vi "Delete Cache.vi"(8 "error in (no error)":errorcluster, 11 "navX Registry Cache in":refnum<class "navX Registry Cache.lvclass">) -> (0 "error out":errorcluster, 2 "Registry Cache":u8[](array[numeric]), 3 "navX Registry Cache out":refnum<class "navX Registry Cache.lvclass">)   [LabVIEW 2015, in "navX Library v3.lvlib" / "navX Registry Cache.lvclass"]
uses:
  navX Registry Cache.lvclass
  navX Registry Cache.lvclass/navX Registry Cache.ctl
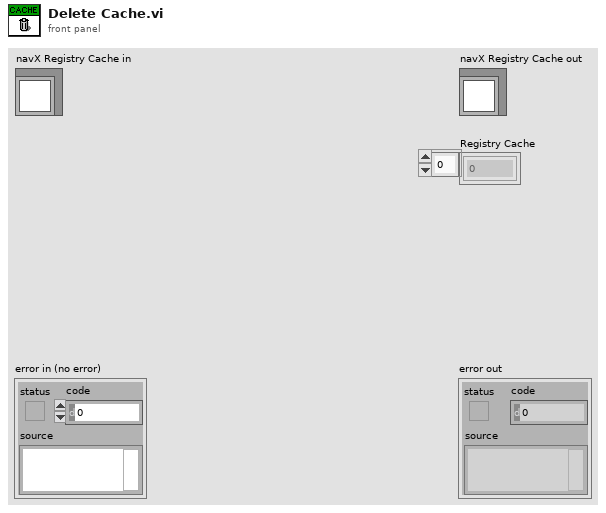
[diagram p1: front panel]
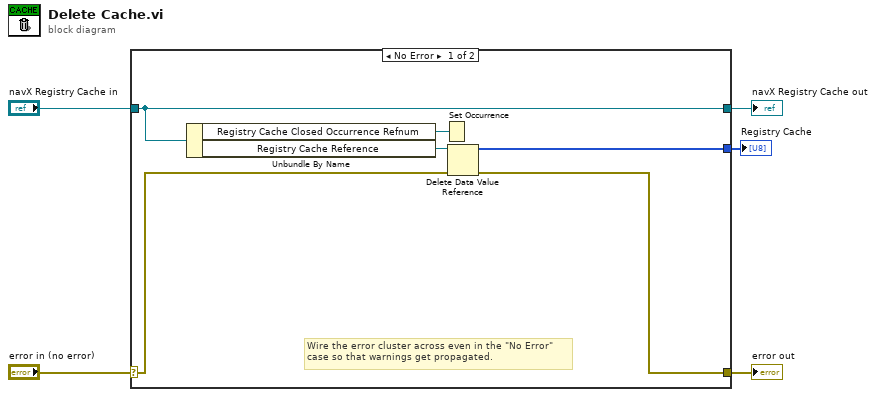
[diagram p0: block diagram]
diagram:
  n1 = case shown="No Error" "error in (no error)" {
    selector: "error in (no error)" -> [w9 w13]
    tunnel: [w8 w13] -> w4
    tunnel: [w11 w12] -> w2
    tunnel: "navX Registry Cache in" -> [w11 w12]
    tunnel: [w7 _] -> w1
    frame No Error {
      # "Wire the error cluster across even in the \"No Error\"\ncase so that warnings get propagated."
      n2 = Unbundle By Name(w11) -> ("Registry Cache Closed Occurrence Refnum"=w6:refnum<k4>, "Registry Cache Reference"=w10:refnum<data-value>)
      n3 = Set Occurrence(w6) -> ()
      n4 = Delete Data Value Reference(data value reference=w10, error in=w9) -> (data value=w7:u8[], error out=w8:errorcluster)
    }
    frame Error {
    }
  }
  "error out" <- w4
  "navX Registry Cache out" <- w2
  "Registry Cache" <- w1
